vi "blockdiagram.vi"   [LabVIEW 2018]
uses:
  <vilib>/Analysis/_algsub.llb/Matrix Norm Type.ctl
  <vilib>/Analysis/_algsub.llb/Real Matrix Norm.vi
  <vilib>/addons/Control Design/_Model Construction/Model Creation.llb/Model Creation SubVI/cd_Create Transfer Function Model.vi
  <vilib>/addons/Control Design/_Model Conversions/Continuous and Discrete.llb/Continuous and Discrete SubVI/cd_Convert Continuous to Discrete (TF).vi
  <vilib>/addons/Control Design/_Model Conversions/Model Type.llb/Model Conversion SubVI/cd_Convert Transfer Function to State-Space Model.vi
  <vilib>/imath/engines/lvmath/Plug In/Control Design/BuiltInFunctions/ss/NIMS_CD_ss(A,B,C,D).vi
  <vilib>/imath/engines/lvmath/Plug In/Control Design/BuiltInFunctions/step/NIMS_CD_[Y,T,X]=step(SS,[Tinfo]).vi
  <vilib>/imath/engines/lvmath2/RunTimeEngine/IndexReplace/NIMS M(S)=S.vi
  <instcachedir>/0/NIMS M(S)=S_3A43114EBE4B4893BC108DAA709F76B8.lvgen/NIMS M(S)=S_3A43114EBE4B4893BC108DAA709F76B8_001.vi
  <vilib>/imathl/engines/lvmath/Functions/Error Handling/Create Error.vi
  <vilib>/imath/engines/lvmath2/RunTimeSupport/NIMS_Get Any Vector_w Error - Matrix.vi
  <instcachedir>/0/NIMS_Get Any Vector_w Error - Matrix_1B26302039EC43C7B9FA287B1E12D88C.lvgen/NIMS_Get Any Vector_w Error - Matrix_1B26302039EC43C7B9FA287B1E12D88C_001.vi
  <vilib>/imath/engines/lvmath2/RunTimeEngine/BuiltInFunctions/toeplitz/NIMS_toeplitz(GV,GV).vi
  <instcachedir>/0/NIMS_toeplitz(GV,GV)_904A8CA474F04DBD8735AC4A531FF7A7.lvgen/NIMS_toeplitz(GV,GV)_904A8CA474F04DBD8735AC4A531FF7A7_002.vi
  <vilib>/imath/engines/lvmath2/RunTimeEngine/ErrorHandling/NIMS_Create Error From Enums.vi
  <vilib>/imath/engines/lvmath2/RunTimeEngine/RangeToken/NIMS_Range.vi
  <instcachedir>/0/NIMS_Range_846134F467D14A349F7C6CCEF459CDB2.lvgen/NIMS_Range_846134F467D14A349F7C6CCEF459CDB2_000.vi
  <vilib>/imath/engines/lvmath2/RunTimeEngine/BuiltInFunctions/eye/NIMS_M=eye(I32).vi
  <vilib>/imath/engines/lvmath2/RunTimeEngine/NodeEndStatement/NIMS_NodeEndStatement_Output.vi
  <instcachedir>/0/NIMS_NodeEndStatement_Output_53EC0D466D134D7ABD903AC30B43404B.lvgen/NIMS_NodeEndStatement_Output_53EC0D466D134D7ABD903AC30B43404B_005.vi
  <instcachedir>/0/NIMS_NodeEndStatement_Output_53EC0D466D134D7ABD903AC30B43404B.lvgen/NIMS_NodeEndStatement_Output_53EC0D466D134D7ABD903AC30B43404B_003.vi
  <instcachedir>/0/NIMS_NodeEndStatement_Output_53EC0D466D134D7ABD903AC30B43404B.lvgen/NIMS_NodeEndStatement_Output_53EC0D466D134D7ABD903AC30B43404B_000.vi
  <vilib>/imath/engines/lvmath2/RunTimeEngine/ErrorHandling/NIMS_Finalize Error.vi
  <vilib>/imath/engines/lvmath2/RunTimeEngine/ArithmeticOperatorToken/NIMS_ArithmeticOperator_multmx.vi
  <instcachedir>/0/NIMS_ArithmeticOperator_multmx_622CA76F9646436AB036D42A9A1CE0E6.lvgen/NIMS_ArithmeticOperator_multmx_622CA76F9646436AB036D42A9A1CE0E6_003.vi
  <vilib>/imath/engines/lvmath2/RunTimeEngine/ArithmeticOperatorToken/NIMS_ArithmeticOperator_minus.vi
  <instcachedir>/0/NIMS_ArithmeticOperator_minus_C4D0373119CC411691B2E50DF2E09F22.lvgen/NIMS_ArithmeticOperator_minus_C4D0373119CC411691B2E50DF2E09F22_009.vi
  <vilib>/imath/engines/lvmath2/RunTimeEngine/RangeToken/NIMS_Range_R2 - Integer.vi
  <instcachedir>/0/NIMS_Range_R2 - Integer_E35B921DECF84AADB7325A02D418BFCC.lvgen/NIMS_Range_R2 - Integer_E35B921DECF84AADB7325A02D418BFCC_000.vi
  <vilib>/imath/engines/lvmath2/RunTimeEngine/CommandStatement/MC_CommandStatement_break.vi
  <vilib>/imath/engines/lvmath2/RunTimeEngine/VariableToken/NIMS_VariableToken_CondDefinedDefinedByReplace.vi
  <instcachedir>/0/NIMS_VariableToken_CondDefinedDefinedByReplace_D162CFFC24174562A9FEA619A91E1A56.lvgen/NIMS_VariableToken_CondDefinedDefinedByReplace_D162CFFC24174562A9FEA619A91E1A56_002.vi
  <vilib>/imath/engines/lvmath2/RunTimeEngine/BuiltInFunctions/norm/NIMS_norm(GM,DBL).vi
  <instcachedir>/0/NIMS_norm(GM,DBL)_14A9435485184B5E92336AF75A728284.lvgen/NIMS_norm(GM,DBL)_14A9435485184B5E92336AF75A728284_001.vi
  <vilib>/imath/engines/lvmath2/RunTimeEngine/IndexReplace/NIMS V(S)=S.vi
  <instcachedir>/0/NIMS V(S)=S_420DA4522869420292A92FA3CC108C4E.lvgen/NIMS V(S)=S_420DA4522869420292A92FA3CC108C4E_000.vi
  <vilib>/imath/engines/lvmath2/RunTimeEngine/IndexRead/NIMS V(S).vi
  <instcachedir>/0/NIMS V(S)_0488751826AF41519A22953C041130DC.lvgen/NIMS V(S)_0488751826AF41519A22953C041130DC_000.vi
  <vilib>/imath/engines/lvmath2/RunTimeEngine/ArithmeticOperatorToken/NIMS_ArithmeticOperator_plus.vi
  <instcachedir>/0/NIMS_ArithmeticOperator_plus_DE670E32103C4C10ADF2A97367172B30.lvgen/NIMS_ArithmeticOperator_plus_DE670E32103C4C10ADF2A97367172B30_002.vi
  <vilib>/imath/engines/lvmath2/RunTimeEngine/NodeEndStatement/NIMS_NodeEndStatement_Get Vector.vi
  <instcachedir>/0/NIMS_NodeEndStatement_Get Vector_329D0992E87F49F089135171B7FC9327.lvgen/NIMS_NodeEndStatement_Get Vector_329D0992E87F49F089135171B7FC9327_003.vi
  <vilib>/imath/engines/lvmath2/RunTimeEngine/VariableToken/NIMS_VariableToken_CondDefined.vi
  <instcachedir>/0/NIMS_VariableToken_CondDefined_BADDB804EBCA4B86883699DABD34B224.lvgen/NIMS_VariableToken_CondDefined_BADDB804EBCA4B86883699DABD34B224_002.vi
  <vilib>/Analysis/Matrix/Numeric/Conversions/Array To Matrix - RA2.vi
  <vilib>/imath/engines/lvmath/Functions/Error Handling/MergeErrorsWrapper.vi
  <instcachedir>/0/NIMS_NodeEndStatement_Output_53EC0D466D134D7ABD903AC30B43404B.lvgen/NIMS_NodeEndStatement_Output_53EC0D466D134D7ABD903AC30B43404B_010.vi
  <vilib>/addons/Control Design/_Model Conversions/NI_CD_Model Type.lvlib
  <vilib>/addons/Control Design/_Model Conversions/NI_CD_Continuous and Discrete.lvlib
  <vilib>/Analysis/NI_AALPro.lvlib
  <vilib>/addons/Control Design/_Model Construction/NI_LinSys_Model Creation.lvlib
  <vilib>/Analysis/Matrix/NI_Matrix.lvlib
types:
  T1 = typedef "NI_AALPro.lvlib/Matrix Norm Type.ctl" = i32
  T2 = typedef "NI_LinSys_Model Typedefs.lvlib/CD Transfer Function Model (MIMO).ctl" = cluster{"properties":T3, "transfer function(s)":T4[][]}
  T3 = typedef "NI_LinSys_Model Typedefs.lvlib/CD General Elements.ctl" = cluster{"Model name":string, "Input names":string[], "Output names":string[], "Input Delays":dbl[], "Output Delays":dbl[], "Sampling Time":dbl, "Notes":string}
  T4 = typedef "NI_LinSys_Model Typedefs.lvlib/CD Transfer Function Model (SISO).ctl" = cluster{"Numerator":dbl[], "Denominator":dbl[], "delay":dbl}
  T5 = typedef "NI_LinSys_Model Typedefs.lvlib/CD State Space Model (MIMO).ctl" = cluster{"properties":T3, "A":dbl[][], "B":dbl[][], "C":dbl[][], "D":dbl[][], "StateNames":string[], "Transport Delay":dbl[][]}
  T6 = typedef "NI_Matrix.lvlib/RealMatrix.ctl" = dbl[][]
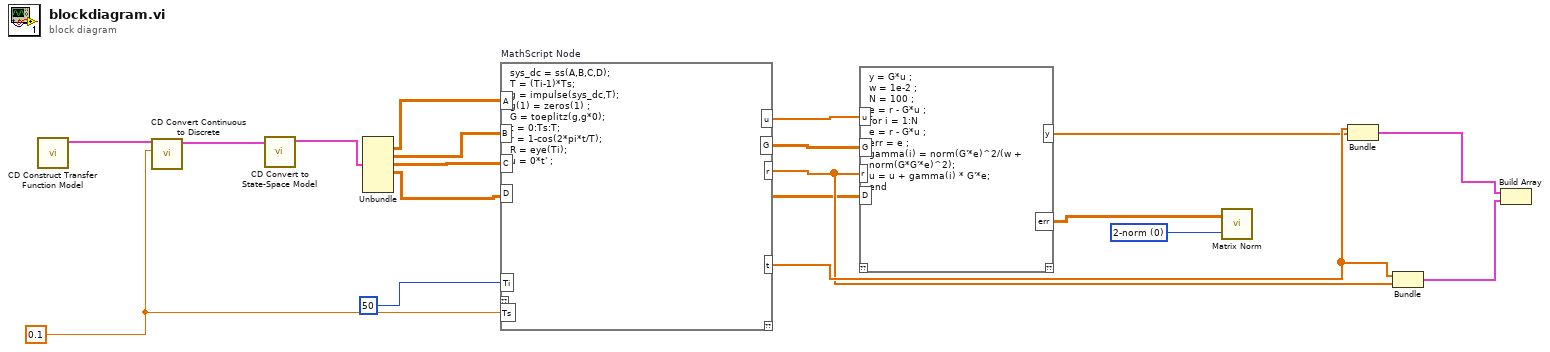
[diagram p0: block diagram]
diagram:
  w10 = T1 0 items=["2-norm", "1-norm", "F-norm", "Inf-norm"] ("norm type")
  w17 = 0.1
  n1 = call-poly <vilib>:"CD Construct Transfer Function Model.vi"() -> ("Transfer Function Model"=w3:T2)  [unwired: 10 in, 1 out]
  n2 = call-poly <vilib>:"CD Convert Continuous to Discrete.vi"("Sampling Time (s)"=w17, "Continuous Transfer Function Model"=w3) -> ("Discrete Transfer Function Model"=w16:T2)  [unwired: 8 in, 1 out]
  n3 = call-poly <vilib>:"CD Convert to State-Space Model.vi"("Transfer Function Model"=w16) -> ("State-Space Model"=w15:T5)  [unwired: 9 in, 1 out]
  n4 = Unbundle "Unbundle"(w15) -> ("A"=w5:dbl[][], "B"=w14:dbl[][], "C"=w13:dbl[][], "D"=w4:dbl[][])  [unwired: 3 out]
  n5 = mathscript code="sys_dc = ss(A,B,C,D);\nT = (Ti-1)*Ts;\ng = impulse(sys_dc,T);\ng(1) = zeros(1) ;\nG = toeplitz(g,g*0);\nt = 0:Ts:T;\nr = 1-cos(2*pi*t/T);\nR = eye(Ti);\nu = 0*t' ;"("Ts"=w17, "Ti"=50, "A"=w5, "B"=w14, "C"=w13, "D"=w4) -> ("u"=w12:cdb[], "G"=w11:cdb[][], "r"=w8:dbl[], "t"=w9:dbl[])  [unwired: 1 in, 1 out]
  n6 = mathscript code="y = G*u ;\nw = 1e-2 ;\nN = 100 ;\ne = r - G*u ;\nfor i = 1:N \ne = r - G*u ;\nerr = e ;\ngamma(i) = norm(G'*e)^2/(w + norm(G*G'*e)^2);\nu = u + gamma(i) * G'*e;\nend"("u"=w12, "G"=w11, "r"=w8, "D"=w4) -> ("err"=w2:T6, "y"=w1:cdb[])  [unwired: 1 in, 1 out]
  n7 = call-poly <vilib>:"Matrix Norm.vi"("norm type"=w10, "Input Matrix"=w2) -> ()  [unwired: 2 out]
  n8 = Bundle("t"=w9, "y"=w1) -> (w7:cluster{"t":dbl[], "y":cdb[]})  [unwired: 1 in]
  n9 = Bundle("t"=w9, "r"=w8) -> (w6:cluster{"t":dbl[], "r":dbl[]})  [unwired: 1 in]
  n10 = Build Array(w7, w6) -> ()  [unwired: 1 out]
